vi "Write to Hardware.vi"(7 "Valid Triggers":bool, 8 "error in (no error)":errorcluster, 9 "Trigger Values":dbl[](array[numeric]), 10 "Values in":dbl[](array[numeric]), 11 "Execution Unit Implementation in":refnum<class "Execution Unit.lvclass">) -> (0 "error out":errorcluster, 1 "Trigger Values out":dbl[](array[numeric]), 2 "Values out":dbl[](array[numeric]), 3 "Execution Unit Implementation out":refnum<class "Execution Unit.lvclass">)   [LabVIEW 2020, in "AIM ARINC 664 Engine.lvlib" / "Implementation.lvlib" / "Execution Unit.lvclass"]
uses:
  Execution Unit.lvclass
  Execution Unit.lvclass/Execution Unit.ctl
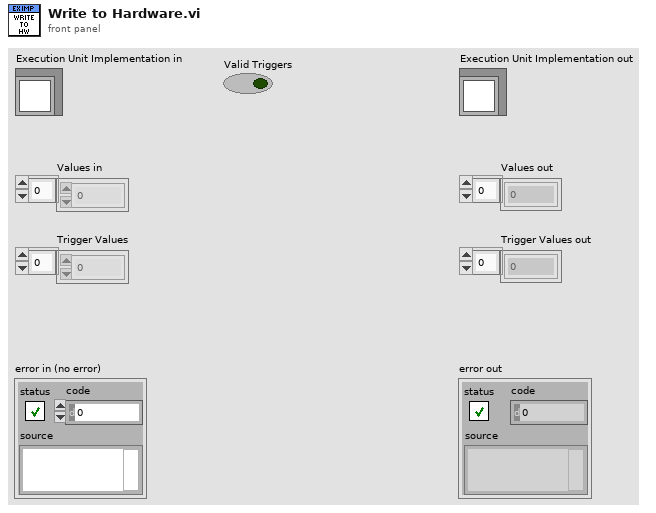
[diagram p1: front panel]
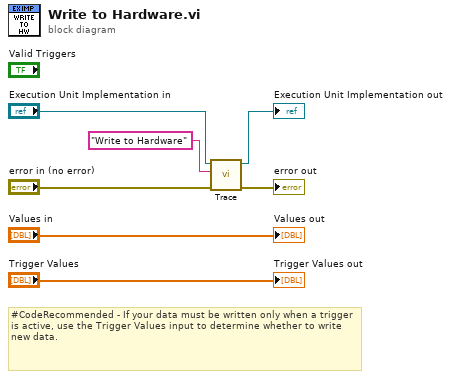
[diagram p0: block diagram]
diagram:
  # "#CodeRecommended - If your data must be written only when a trigger is active, use the Trigger Values input to determine whether to write new data."
  n1 = call "Trace.vi"("Execution Unit Implementation in"="Execution Unit Implementation in", "message"="Write to Hardware", "error in (no error)"="error in (no error)") -> ("Execution Unit Implementation out"=→"Execution Unit Implementation out":refnum<class "Execution Unit.lvclass">, "error out"=→"error out":errorcluster)  [unwired: 6 in]
  "Values out" <- "Values in"
  "Trigger Values out" <- "Trigger Values"
